vi "niRFUtil RFHS Apply Polynomial DPD using LUT (complex array).vi"(0 "x[n]":csg[](array[numeric]) format="%.2f", 1 "|x[n]|":sgl[](array[numeric]) min=0 max=127 format="%.2f", 2 "f(x)":csg[](array[numeric]) format="%.2f", 3 "x.start":sgl, 4 "x.step":sgl, 5 "error in":errorcluster) -> (14 "x[n].f(|x[n]|)":csg[](array[numeric]), 19 "error out":errorcluster)   [LabVIEW 2015, in "niRFUtil.lvlib"]
uses:
  niRFUtil.lvlib
panel:
  out "AVX":csg[](array[numeric])
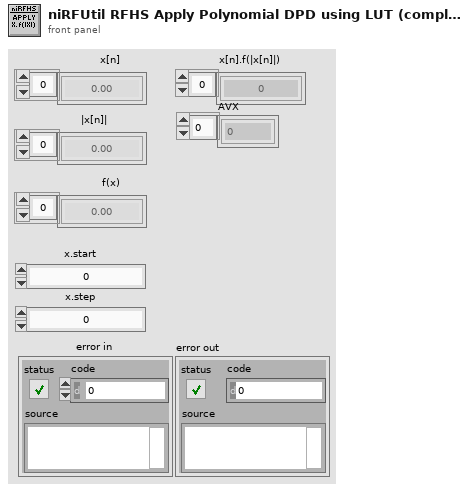
[diagram p1: front panel]
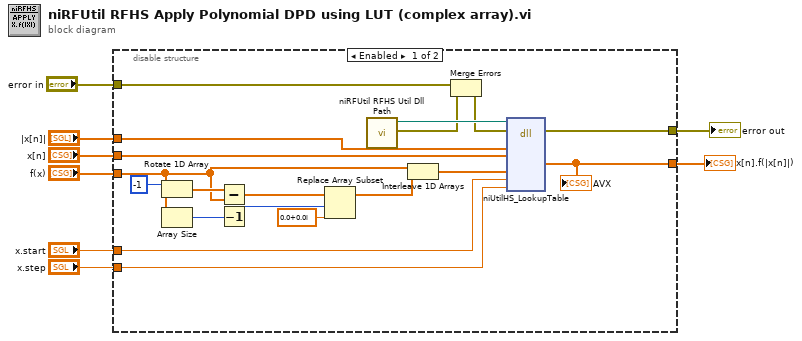
[diagram p0: block diagram]
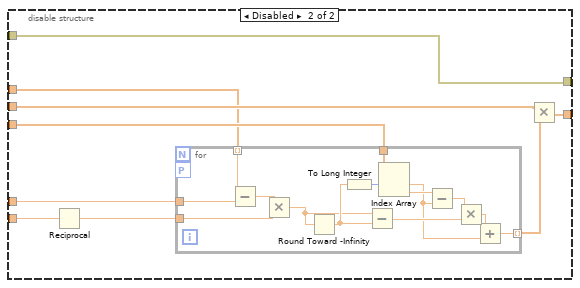
[diagram p2: hidden frame]
diagram:
  n1 = disable-structure shown="Enabled" {
    disable-tunnel: [w18 w32] -> w8
    disable-tunnel: "x[n]" -> [w17 w33]
    disable-tunnel: "|x[n]|" -> [w16 w30]
    disable-tunnel: "x.start" -> [w15 w29]
    disable-tunnel: "x.step" -> [w14 w35]
    disable-tunnel: "f(x)" -> [w13 w36]
    disable-tunnel: [w12 w31] -> w2
    disable-tunnel: "error in" -> [w11 w31]
    frame Enabled {
      n2 = Rotate 1D Array(1:w13, 2:-1 ("n")) -> (0:w26:csg[])
      n3 = Array Size(array=w13) -> (size(s)=w23:i32)
      n4 = Subtract(x=w26, y=w13) -> (x-y=w25:csg[])
      n5 = Decrement(x=w23) -> (x-1=w24:i32)
      n6 = Replace Array Subset(array=w25, new element=csg 0.0+0.0i ("new element/subarray"), index=w24) -> (w21:csg[])
      n7 = call "niRFUtil RFHS Util Dll Path.vi"() -> ("error out"=w10:errorcluster, "Path"=w19:path)  [unwired: 7 in, 3 out]
      n8 = Interleave 1D Arrays(w13, w21) -> (w20:csg[])
      n9 = Merge Errors(w11, w10) -> (w9:errorcluster)
      n10 = dll-call lib="niRFHS_avx.*" fn="niUtilHS_LookupTable"(path in=w19, error in=w9, "iBuf"=w16, "iWav"=w17, "LUTData"=w20, "a"=w15, "b"=w14) -> (error out=w12:errorcluster, "AVX"=w18:csg[])  [unwired: 8 in, 1 out]
      "AVX" <- w18
    }
    frame Disabled {
      n11 = Reciprocal(x=w35) -> (1/x=w28:sgl)
      n12 = for {
        tunnel: w36 -> [w45]
        tunnel: [w44] -> w34 mode=indexing
        workers-P: _ -> [_]
        tunnel: w30 -> [w40] mode=indexing
        tunnel: w29 -> [w39]
        tunnel: w28 -> [w38]
        n13 = Subtract(x=w40, y=w39) -> (x-y=w41:sgl)
        n14 = Multiply(x=w41, y=w38) -> (x*y=w37:sgl)
        n15 = Round Toward -Infinity(1:w37) -> (0:w42:sgl)
        n16 = To Long Integer(number=w42) -> (32bit integer=w43:i32)
        n17 = Subtract(x=w37, y=w42) -> (x-y=w48:sgl)
        n18 = Index Array(array=w45, index #1=w43) -> (element #1=w46:csg, element #2=w50:csg)  [unwired: 1 in]
        n19 = Subtract(x=w50, y=w46) -> (x-y=w49:csg)
        n20 = Multiply(x=w49, y=w48) -> (x*y=w47:csg)
        n21 = Add(x=w47, y=w46) -> (x+y=w44:csg)
      }
      n22 = Multiply(x=w33, y=w34) -> (x*y=w32:csg[])
    }
  }
  "x[n].f(|x[n]|)" <- w8
  "error out" <- w2
